vi "bremsmoment.vi"(11 "Dynamic Data in":dynamicdata(waveform)) -> (3 "Dynamic Data out":dynamicdata(waveform))   [LabVIEW 2018]
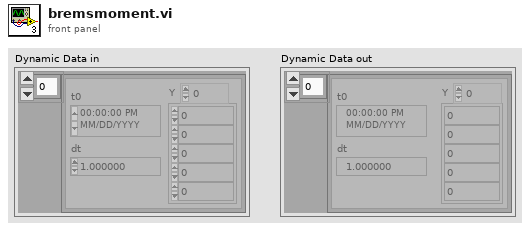
[diagram p1: front panel]
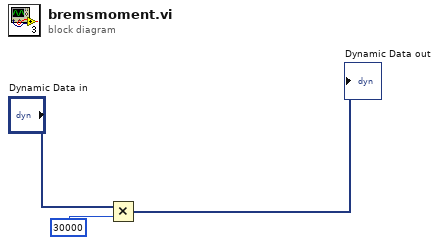
[diagram p0: block diagram]
diagram:
  n1 = Multiply(x="Dynamic Data in", y=30000) -> (x*y=→"Dynamic Data out":dynamicdata)
